vi "MG FileName.vi"(8 "Fehler (Eingang)":errorcluster, 10 "Gasnummer:":u8, 11 "Lin-Polynom":T1 {"zusätzliche Zeitdauer Erster Punkt" format="%#_5g"; "Lin Modus" items=["Cal Gas to PNS", "Cal Gas to Samplepoint", "Measure"]; "Gas Ablaufdatum" format="%<%d.%m.%Y>T"; "HovaCAL Flow AutoLin"."HovaCAL Flow Input Cluster" format="%.2f"; "Gasflasche" items=["----"=10000, "IAG MG"=0, "IAG NH3 3000"=1, "IAG NH3 2000"=2, "IAG NH3 200"=3]; "Conditions:" items=["field", "laboratory"]; "Kalibrierauswahl" items=["Inaktiv", "Aktiv"]; "Anzahl Stufen" format="%#_5g"; "Zeitdauer Stufe" format="%#_5g"; "Verdünnungsgas" items=["N2", "O2"]; "Komponentenauswahl"."Konzentration" format="%#.6f"; "Gasnummer:" min=1 max=5; "Prüfgas Konzentration" format="%#.6f"; "Polynomkoeff." format="%#_18f"}) -> (0 "Fehler (Ausgang)":errorcluster, 2 "LIN TXT Datei Name":string, 3 "EPA TXT Datei Name":string, 5 "MG Name":string)   [LabVIEW 2020, in "Linearisierung v2.lvlib"]
uses:
  Linearisierung v2.lvlib
  Lin-Polynom Daten.ctl
  KomponentenArray.ctl
  Visualisierungs Elemente/Auswahlfeld.ctl
  Visualisierungs Elemente/Zahlen-Eingabefeld.ctl
  EPA Optionsfeld.ctl
  Gasteiler/HovaCal/AutoLin Hovacal.ctl
  Kalibrieroption.ctl
  EPA1065-307/Condition.ctl
  Seiten/System Einstellungen V2/Konfig Gasflasche.ctl
  Seiten/System Einstellungen V2/Gasflasche Auswahl.ctl
  Gasteiler/HovaCAL_Interface/Controls/Flow Einstellung.ctl
  Gasteiler/HovaCAL_Interface/Controls/Pump state.ctl
  Seiten/CalGas Aufschaltung/Lin Modus.ctl
  Visualisierungs Elemente/String - Ausgabefeld.ctl
  SpanEinstellungen/Aktion FGV SpanEinstellungen.ctl
  Seiten/FT-IR/FGV FT-IR Gasliste Aktionen.ctl
  Gasteiler/Aktion FGV Gasteilerliste laden.ctl
  Gasteiler/Gasteiler.lvlib
  Seiten/FT-IR/FT-IR.lvlib
  SpanEinstellungen/SpanEinstellungen.lvlib
  Gasteiler/HovaCal/HovaCal.lvlib
  EPA1065-307/Linearity verification 1065-307.lvlib
  Seiten/System Einstellungen V2/System Einstellungen V2.lvlib
  Gasteiler/HovaCAL_Interface/Controls/Controls.lvlib
  Seiten/CalGas Aufschaltung/CalGas Aufschaltung.lvlib
panel:
  # "%"
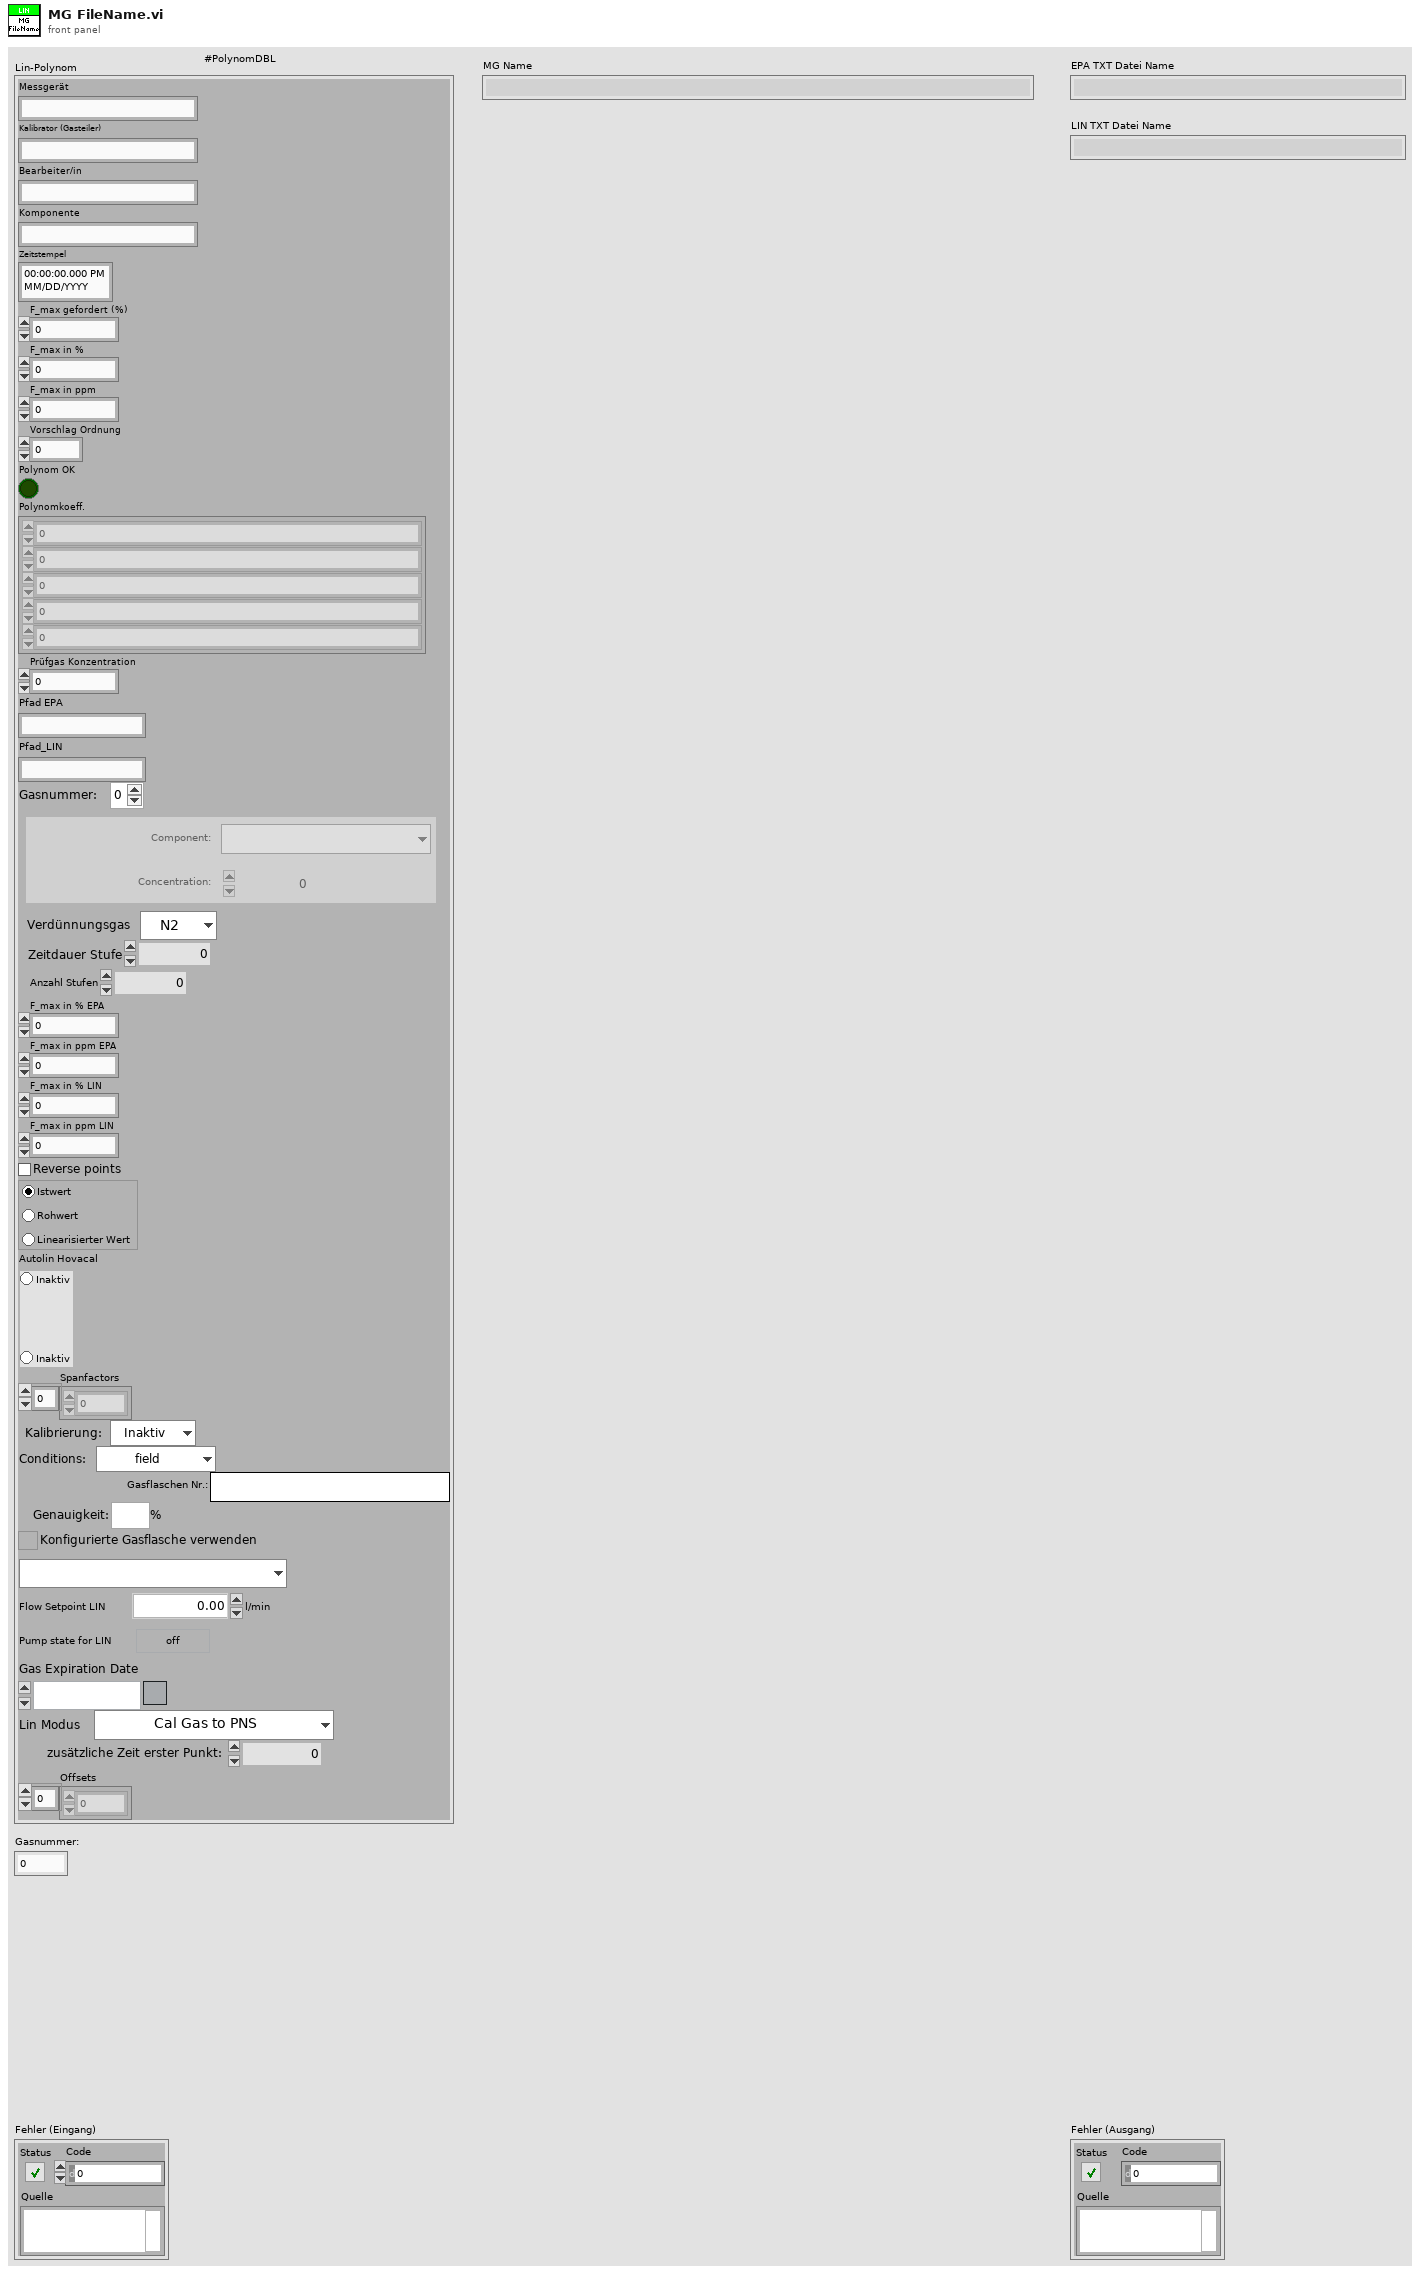
[diagram p1: front panel]
types:
  T1 = typedef "Linearisierung v2.lvlib/Lin-Polynom Daten.ctl" = cluster{"Messgerät":string, "Kalibrator (Gasteiler)":string, "Bearbeiter/in":string, "Komponente":string, "Zeitstempel":timestamp, "F_max gefordert (%)":sgl, "F_max in %":sgl, "F_max in ppm":sgl, "Vorschlag Ordnung":i32, "Polynom OK":bool, "Polynomkoeff.":dbl[], "Prüfgas Konzentration":dbl, "Pfad EPA":string, "Pfad_LIN":string, "Gasnummer:":u8, "Komponentenauswahl":T2, "Verdünnungsgas":T4, "Zeitdauer Stufe":T5, "Anzahl Stufen":T5, "F_max in % EPA":sgl, "F_max in ppm EPA":sgl, "F_max in % LIN":sgl, "F_max in ppm LIN":sgl, "Punkte umkehren":bool, "EPA Optionsfeld":T6, "Autolin Hovacal":T7, "Spanfactors":sgl[], "Kalibrierauswahl":T8, "Conditions:":T9, "Gasflaschen Nr.:":string, "Bottle Accuracy":dbl, "Konfig Gasflasche":T10, "Gasflasche":T11, "HovaCAL Flow AutoLin":T12, "MFC Output":T13, "Gas Ablaufdatum":timestamp, "Lin Modus":T14, "zusätzliche Zeitdauer Erster Punkt":sgl, "Offsets":sgl[]}
  T2 = typedef "Linearisierung v2.lvlib/KomponentenArray.ctl" = cluster{"Komponente:":T3, "Konzentration":dbl}[]
  T3 = typedef "Auswahlfeld.ctl" = u16
  T4 = typedef "Linearisierung v2.lvlib/Gasteiler.lvlib/Prüfgas in.ctl" = u16
  T5 = typedef "Zahlen-Eingabefeld.ctl" = sgl
  T6 = typedef "Linearisierung v2.lvlib/EPA Optionsfeld.ctl" = enum32{"Istwert", "Rohwert", "Linearisierter Wert"}
  T7 = typedef "Linearisierung v2.lvlib/Gasteiler.lvlib/HovaCal.lvlib/AutoLin Hovacal.ctl" = enum32{"Keine Auswahl", "Optionsauswahl 1", "Optionsauswahl 2"}
  T8 = typedef "Linearisierung v2.lvlib/Kalibrieroption.ctl" = u16
  T9 = typedef "Linearisierung v2.lvlib/Linearity verification 1065-307.lvlib/Condition.ctl" = u16
  T10 = typedef "System Einstellungen V2.lvlib/Konfig Gasflasche.ctl" = bool
  T11 = typedef "System Einstellungen V2.lvlib/Gasflasche Auswahl.ctl" = u16
  T12 = typedef "Linearisierung v2.lvlib/Gasteiler.lvlib/HovaCAL_Interface.lvlib/Controls.lvlib/Flow Einstellung.ctl" = cluster{"HovaCAL Flow Input Cluster":dbl}
  T13 = typedef "Linearisierung v2.lvlib/Gasteiler.lvlib/HovaCAL_Interface.lvlib/Controls.lvlib/Pump state.ctl" = cluster{"Run":bool}
  T14 = typedef "CalGas Aufschaltung.lvlib/Lin Modus.ctl" = u16
  T15 = typedef "Linearisierung v2.lvlib/SpanEinstellungen.lvlib/Aktion FGV SpanEinstellungen.ctl" = enum16{"lesen", "schreiben", "laden", "speichern", "RegisterRef", "automatisch", "init", "PDF Params", "Punkte umkehren"}
  T16 = typedef "String - Ausgabefeld.ctl" = string
  T17 = typedef "Linearisierung v2.lvlib/SpanEinstellungen.lvlib/SpanInletCluster.ctl" = cluster{"Span Inlet Active":T10, "Analysator":T18, "Konfig Gasflasche":T10, "Gasflasche":T11, "Gasflaschen Nr.:":string, "Ablaufdatum":timestamp, "Komponenten":T19, "Zeitdauer Stufen":sgl, "Max Fehler":sgl, "Anzahl Stufen":sgl, "Trägergas":T23, "zusätzliche Zeitdauer Erster Punkt":sgl}
  T18 = typedef "System Einstellungen V2.lvlib/Analysatoren.ctl" = string
  T19 = typedef "Linearisierung v2.lvlib/SpanEinstellungen.lvlib/Komponentencluster mit Formel.ctl" = cluster{"Komponente 1":T20, "Komponente 2":T20, "Komponente 3":T20, "Komponente 4":T20, "Komponente 5":T20}
  T20 = typedef "Linearisierung v2.lvlib/SpanEinstellungen.lvlib/Komponentenauswahl mit Formel.ctl" = cluster{"Komponente:":u16, "Summenformel":T21, "Konzentration IST":dbl, "Einheit":T22, "Genauigkeit":dbl}
  T21 = typedef "String - Eingabefeld.ctl" = string
  T22 = typedef "Linearisierung v2.lvlib/SpanEinstellungen.lvlib/Einheit.ctl" = enum16{"ppm", "%"}
  T23 = typedef "System Einstellungen V2.lvlib/Traegergas.ctl" = string
  T24 = typedef "Linearisierung v2.lvlib/SpanEinstellungen.lvlib/PDF Optionen.ctl" = cluster{"PDF Einzelseiten Komponenten":bool, "PDF Einzelseiten Span":bool, "PDF Deckblatt":bool, "PDF öffnen":bool, "Graphik für Messwerte":bool}
  T25 = cluster{"Punkte umkehren":bool[], "PDF Optionen":T24}
  T26 = typedef "Linearisierung v2.lvlib/Gasteiler.lvlib/Aktion FGV Gasteilerliste laden.ctl" = enum16{"lesen", "laden", "speichern", "Liste erstellen", "Formel ändern", "Gas vereinzeln"}
  T27 = typedef "FT-IR.lvlib/FGV FT-IR Gasliste Aktionen.ctl" = enum16{"lesen", "Gasliste FT-IR", "Gasliste ausgelesen", "laden", "speichern", "löschen"}
  T28 = cluster{"File Name LIN":string, "File Name EPA":string, "MG":bool}
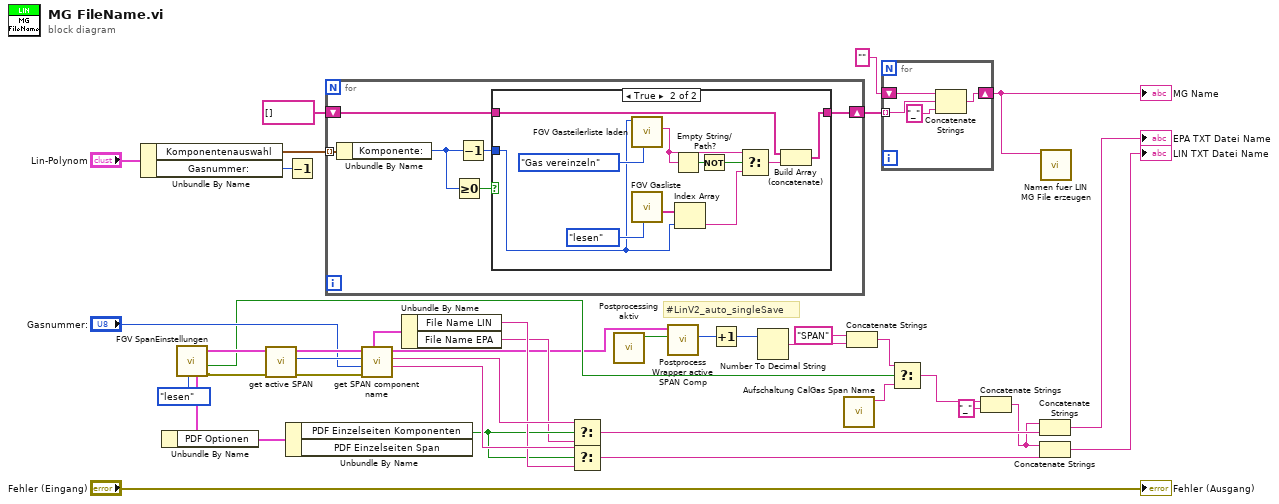
[diagram p0: block diagram]
diagram:
  # "#LinV2_auto_singleSave"
  n1 = Unbundle By Name("Lin-Polynom") -> ("Komponentenauswahl"=w36:T2, "Gasnummer:"=w28:u8)
  n2 = call "FGV SpanEinstellungen.vi"("Aktion"=Aktion_FGV_SpanEinstellungen."lesen") -> ("error out"=w32:errorcluster, "automatisch out"=w10:T10, "SpanInletClusterArray out"=w33:T17[], "Punkte umkehren und PDF Optionen Cluster"=w14:T25)  [unwired: 6 in, 1 out]
  n3 = Unbundle By Name(w14) -> ("PDF Optionen"=w13:T24)
  n4 = call "get active SPAN.vi"("error in (no error)"=w32, "SpanInletClusterArray in"=w33) -> ("error out"=w30:errorcluster, "Index active SPAN"=w29:i32, "SpanInletClusterArray out"=w31:T17[])  [unwired: 7 in]
  n5 = Unbundle By Name(w13) -> ("PDF Einzelseiten Komponenten"=w12:bool)  [unwired: 1 out]
  n6 = Decrement(x=w28) -> ()  [unwired: 1 out]
  n7 = for {
    tunnel: w36 -> [w44] mode=indexing
    shift-right: [w45] -> w37
    shift-left: T16[] [] -> [w41]
    n8 = Unbundle By Name(w44) -> ("Komponente:"=w42:T3)
    n9 = Greater Or Equal To 0?(x=w42) -> (x >= 0?=w43:bool)
    n10 = Decrement(x=w42) -> (x-1=w40:T3)
    n11 = case shown="True" w43 {
      tunnel: [w46 w49] -> w45
      tunnel: w40 -> [_ w54]
      tunnel: w41 -> [w46 w48]
      frame False {
      }
      frame True {
        n12 = call "FGV Gasteilerliste laden.vi"("Aktion"=Aktion_FGV_Gasteilerliste_laden."Gas vereinzeln", "Gasindex"=w54) -> ("Formel"=w52:string)  [unwired: 7 in, 2 out]
        n13 = call "FGV Gasliste.vi"("Aktionen"=FGV_FT-IR_Gasliste_Aktionen."lesen") -> ("Aktuelle Gasliste gesamt"=w56:T16[])  [unwired: 8 in, 2 out]
        n14 = Empty String/Path?(string/path=w52) -> (empty?=w53:bool)
        n15 = Index Array(array=w56, index=w54) -> (element=w51:T16)
        n16 = Not(x=w53) -> (.not. x?=w47:bool)
        n17 = Select(t=w52, s=w47, f=w51) -> (s? t:f=w50:T16)
        n18 = Build Array (concatenate)(w48, w50) -> (w49:T16[])
      }
    }
  }
  n19 = call "get SPAN component name.vi"("Fehler (Eingang)"=w30, "Comp Idx"="Gasnummer:", "SPAN Idx"=w29, "SpanInletClusterArray in"=w31) -> ("Protokoll Name LIN"=w23:string, "Protokoll Name EPA"=w24:string, "SpanInletClusterArray out"=w3:T17[], "LIN/EPA TXT Datei Name"=w26:T28)  [unwired: 4 out]
  n20 = Unbundle By Name(w26) -> ("File Name LIN"=w22:string, "File Name EPA"=w11:string)
  n21 = Select(t=w24, s=w12, f=w11) -> (s? t:f=w21:string)
  n22 = Select(t=w23, s=w12, f=w22) -> (s? t:f=w20:string)
  n23 = call "Postprocessing aktiv.vi"() -> ("postprocess"=w4:bool)  [unwired: 10 in, 1 out]
  n24 = call "Postprocess Wrapper active SPAN Comp.vi"("postprocessing"=w4, "SpanInletClusterArray in"=w3) -> ("active reprocessing SPAN"=w2:i32)  [unwired: 6 in, 3 out]
  n25 = Increment(x=w2) -> (x+1=w1:i32)
  n26 = Number To Decimal String(number=w1) -> (decimal integer string=w7:string)  [unwired: 1 in]
  n27 = call "Aufschaltung CalGas Span Name.vi"() -> ("Span Name"=w9:T21)  [unwired: 11 in]
  n28 = Concatenate Strings("SPAN" ("String"), w7) -> (w5:string)
  n29 = for {
    tunnel: w37 -> [w61] mode=indexing
    shift-right: [w58] -> w27
    shift-left: "" -> [w59]
    n30 = Concatenate Strings(w59, w61, "_") -> (w58:string)
  }
  "MG Name" <- w27
  n31 = Select(t=w5, s=w10, f=w9) -> (s? t:f=w8:T21)
  n32 = Concatenate Strings(w8, "_" ("String")) -> (w18:string)
  n33 = Concatenate Strings(w18, w21) -> (→"EPA TXT Datei Name":string)
  n34 = Concatenate Strings(w18, w20) -> (→"LIN TXT Datei Name":string)
  n35 = call "Namen fuer LIN MG File erzeugen.vi"("String Eingabe"=w27) -> ()  [unwired: 9 in, 2 out]
  "Fehler (Ausgang)" <- "Fehler (Eingang)"
